vi "i2c_controller.vi"(5 "SDA in pin":refnum<k21>="SDA0", 6 "I2C clock divisor":u8=25, 7 "SCL out pin":refnum<k21>="SCL0", 8 "Read FIFO":refnum<k21>="I2C read 0", 9 "Write FIFO":refnum<k21>="I2C write 0", 10 "SDA out pin":refnum<k21>="SDA0", 11 "SCL in pin":refnum<k21>="SCL0") -> ()   [LabVIEW 2011]
uses:
  i2c_controller_state.ctl
  Common/i2c_status.ctl
  <vilib>/Platform/TimedLoop/XDataNode/timing_clust.ctl
  <vilib>/Platform/TimedLoop/XDataNode/nitl_modes.ctl
  <vilib>/Platform/TimedLoop/XDataNode/wakeup.ctl
  <vilib>/rvi/DataTransferAndStorage/Container/Common/niFpgaContainerExecOnDevCompGetState.vi
  <vilib>/rvi/FIFO/Fifo_Resource/nirvififoEmulationSetSize.vi
  <vilib>/rvi/DataTransferAndStorage/Container/Common/niFpgaContainerGetUniqueNameForEmu.vi
  <vilib>/rvi/interface/RandomDataEmulation/nirviRandomDataFPGAFIFO.vi
  <vilib>/rvi/interface/RandomDataEmulation/niFpgaRandomDataHandleErrors.vi
  <vilib>/rvi/eio/common/nirviEmuReportErrorAndStop.vi
  fpga_globals.vi
  <vilib>/Platform/TimedLoop/XDataNode/XDataNode.xnode
  <vilib>/rvi/DataTransferAndStorage/Container/XNode/niFpgaContainer.xnode
  <vilib>/rvi/FIFO/Fifo_Resource/niFpgaFifoEmulationRefIn.vi
  <vilib>/Platform/TimedLoop/XDataNode/XDNodeRunTimeDep.lvlib
panel:
  # "Clock"
  # "I2C bus I/O pins.  The input and output directions  may in general be distinct when an external buffer is used.  See output_buffer.vi"
  # "Data"
  # "Commands and data out to I2C"
  # "Status and data back from I2C"
  # "1/4 of the I2C bit time, in clock ticks"
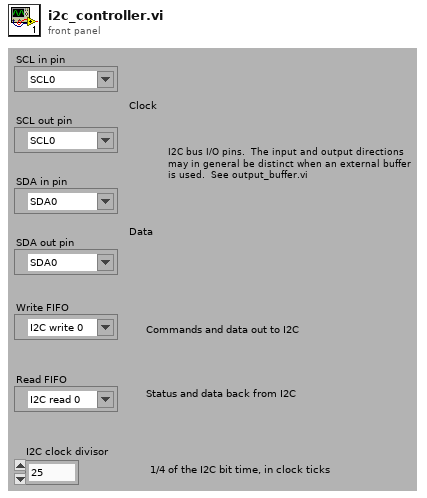
[diagram p1: front panel]
types:
  T1 = typedef "i2c_status.ctl" = enum8{"Invalid", "Command", "I2C start", "Trigger wait", "TX data wait", "Sequence", "Receive data", "I2C error", "Address NACK", "Data NACK", "SDA stuck", "SCL stuck", "Bad command"}
  T2 = typedef "i2c_controller_state.ctl" = enum8{"CMD wait", "start", "load", "address", "address ACK", "wait", "TX data", "TX data ACK", "stop wait", "stop", "RX data", "RX data 1", "RX data ACK", "Sequence arg load", "Trigger delay 1", "Trigger delay 2", "Trigger delay 3"}
  T3 = typedef "XDNodeRunTimeDep.lvlib/timing_clust.ctl" = cluster{"Expected End [f-1]":u64, "Actual End [f-1]":u64, "Finished Late? [f-1]":bool, "Expected End [i-1]":u64, "Actual End [i-1]":u64, "Finished Late? [i-1]":bool, "Expected Start [i]":u64, "Actual Start [i]":u64, "Expected Start [f]":u64, "Actual Start [f]":u64, "Source Name":string, "Structure Name":string, "Period":i64, "Deadline":i64, "Offset":i64, "Start":i64, "Priority":i32, "Timeout":i32, "Mode":T4, "Wakeup Reason":T5, "Error":errorcluster, "Source Type":string, "Secondary Source Type":string, "Global End Time":u64, "Global Start Time":u64, "Frame Duration":u64, "Iteration Duration":u64, "Assigned CPU":i32, "I/O Scan Engine Mode":u32}
  T4 = typedef "XDNodeRunTimeDep.lvlib/nitl_modes.ctl" = enum32{"No Change", "Process missed periods, maintain original phase", "Discard missed periods, maintain original phase", "Process missed periods, ignore original phase", "Discard missed periods, ignore original phase"}
  T5 = typedef "XDNodeRunTimeDep.lvlib/wakeup.ctl" = enum32{"Normal", "Aborted", "Asynchronous wakeup", "Timing source error", "Timed loop error", "Timeout"}
  T6 = typedef "i2c_command.ctl" = enum8{"invalid", "start_write", "start_read", "stop", "sequence"}
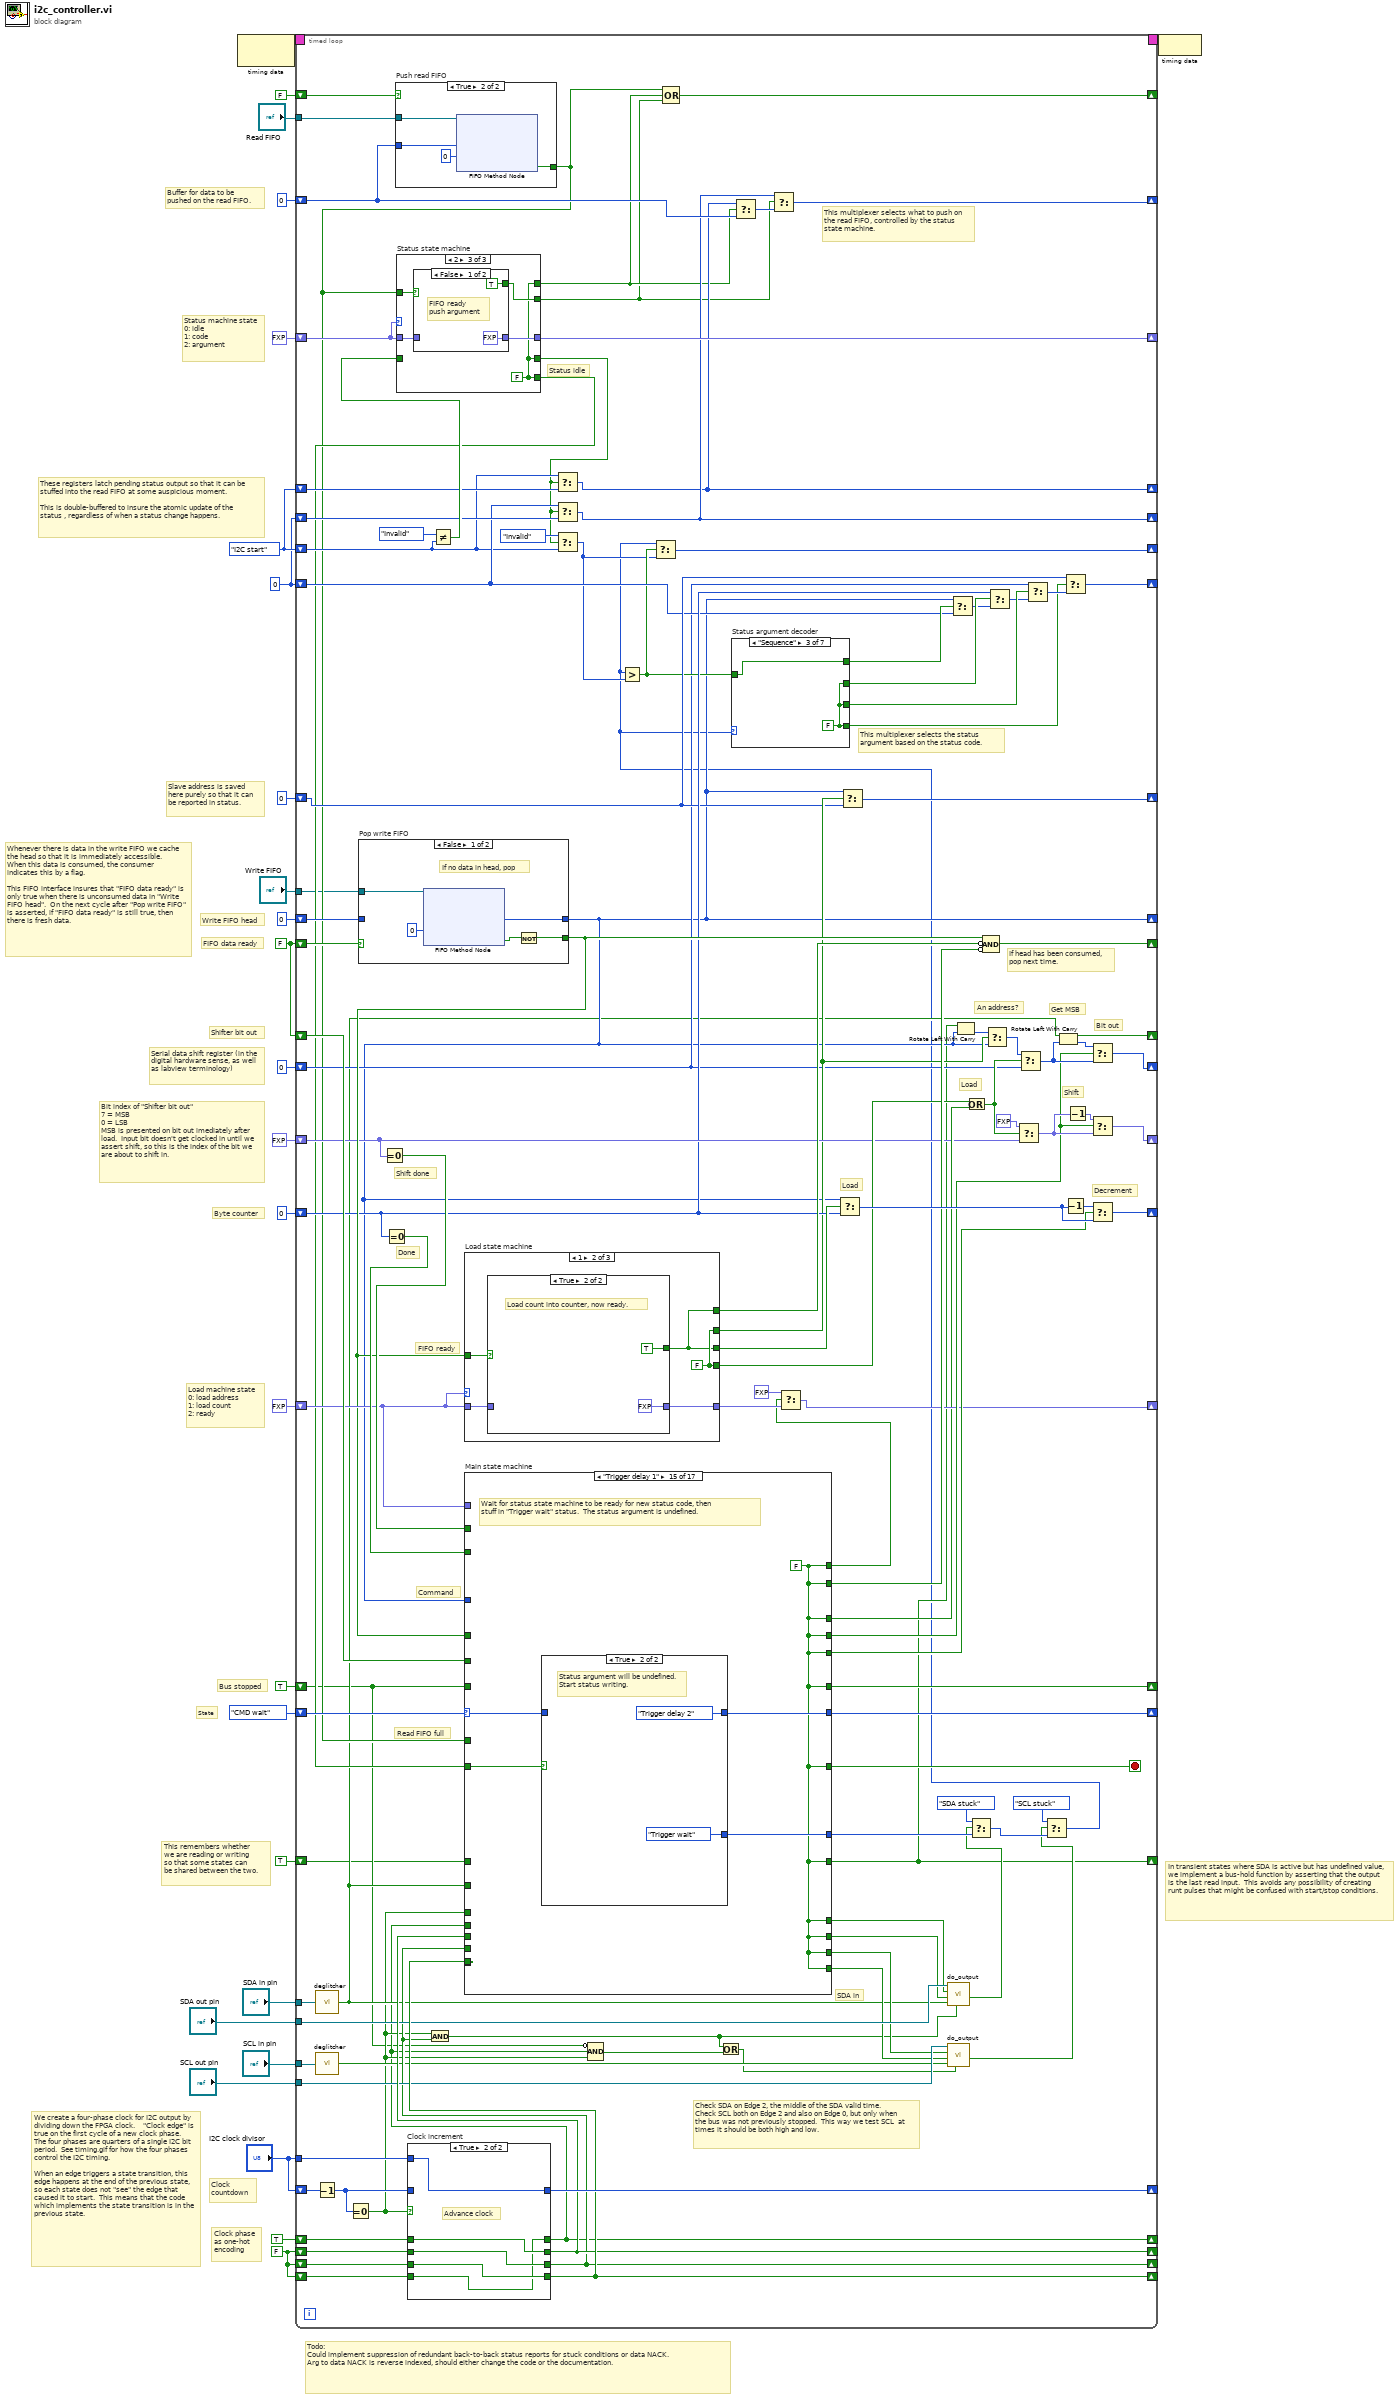
[diagram p0: block diagram]
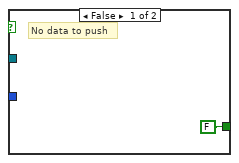
[diagram p2: hidden frame]
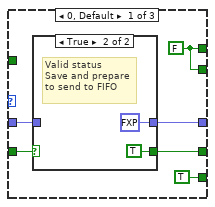
[diagram p3: hidden frame]
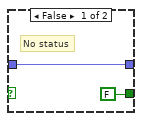
[diagram p4: hidden frame]
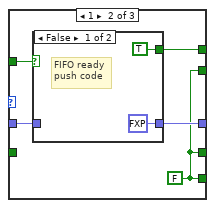
[diagram p5: hidden frame]
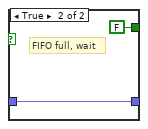
[diagram p6: hidden frame]
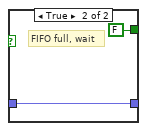
[diagram p7: hidden frame]
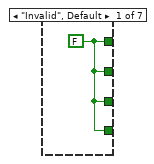
[diagram p8: hidden frame]
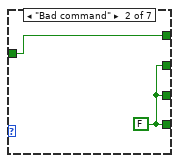
[diagram p9: hidden frame]
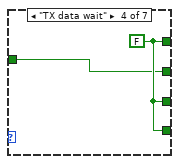
[diagram p10: hidden frame]
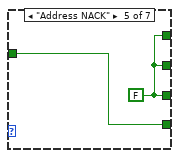
[diagram p11: hidden frame]
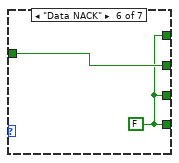
[diagram p12: hidden frame]
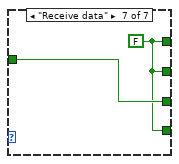
[diagram p13: hidden frame]
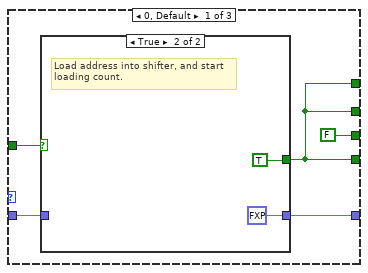
[diagram p14: hidden frame]
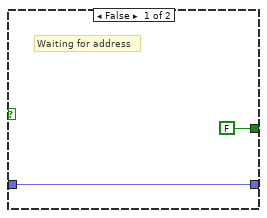
[diagram p15: hidden frame]
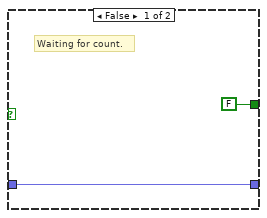
[diagram p16: hidden frame]
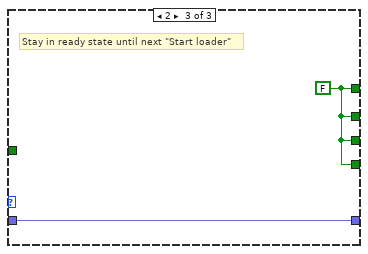
[diagram p17: hidden frame]
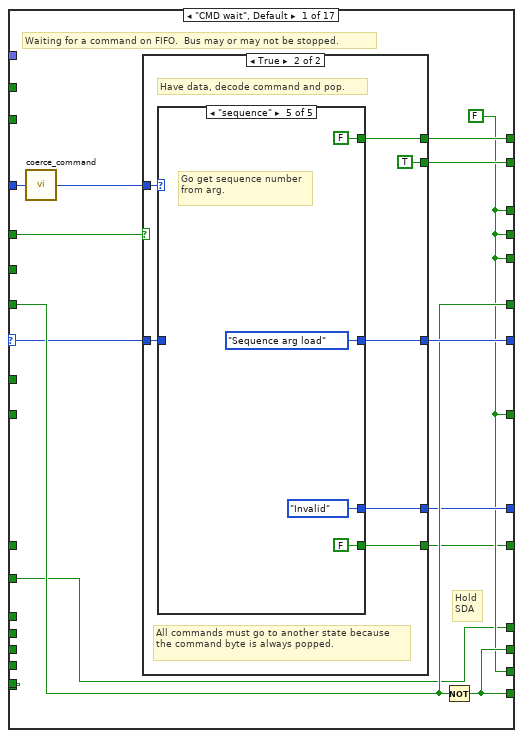
[diagram p18: hidden frame]
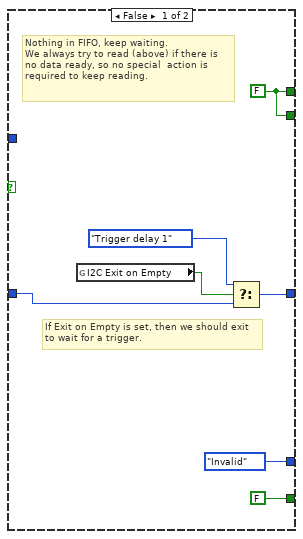
[diagram p19: hidden frame]
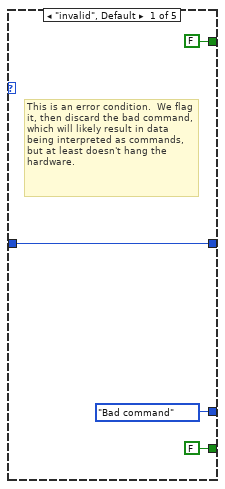
[diagram p20: hidden frame]
diagram:
  w10 = i2c_status."I2C start" ("Cluster")
  w9 = u8 0 ("Element")
  w15 = FALSE ("x = 0?")
  w19 = FALSE
  # "This remembers whether\nwe are reading or writing\nso that some states can\nbe shared between the two."
  # "In transient states where SDA is active but has undefined value, we implement a bus-hold function by asserting that the output is the last read input.  This avoids any possibility of creating runt pulses that might be confused with start/stop conditions."
  # "Buffer for data to be pushed on the read FIFO."
  # "Status machine state\n0: idle\n1: code\n2: argument"
  # "These registers latch pending status output so that it can be stuffed into the read FIFO at some auspicious moment.\n\nThis is double-buffered to insure the atomic update of the status , regardless of when a status change happens."
  # "Slave address is saved here purely so that it can be reported in status."
  # "Todo: \nCould implement suppression of redundant back-to-back status reports for stuck conditions or data NACK.\nArg to data NACK is reverse indexed, should either change the code or the documentation."
  # "Clock phase\nas one-hot\nencoding"
  # "Load machine state\n0: load address\n1: load count\n2: ready"
  # "Bus stopped"
  # "Shifter bit out"
  # "Byte counter"
  # "Serial data shift register (in the digital hardware sense, as well as labview terminology)"
  # "We create a four-phase clock for I2C output by dividing down the FPGA clock.    \"Clock edge\" is true on the first cycle of a new clock phase.  The four phases are quarters of a single I2C bit period.  See timing.gif for how the four phases control the I2C timing.\n\nWhen an edge triggers a state transition, this edge happens at the end of the previous state, so each state does not \"see\" the edge that caused it to start.  This means that the code which implements the state transition is in the previous state."
  # "Whenever there is data in the write FIFO we cache the head so that it is immediately accessible.  When this data is consumed, the consumer indicates this by a flag.\n\nThis FIFO interface insures that \"FIFO data ready\" is only true when there is unconsumed data in \"Write FIFO head\".  On the next cycle after \"Pop write FIFO\" is asserted, if \"FIFO data ready\" is still true, then there is fresh data."
  # "FIFO data ready"
  # "Clock countdown"
  # "Write FIFO head"
  # "State"
  # "Bit index of \"Shifter bit out\"\n7 = MSB\n0 = LSB\nMSB is presented on bit out imediately after load.  Input bit doesn't get clocked in until we assert shift, so this is the index of the bit we are about to shift in."
  n1 = node-c288() -> (w26:T3)  [unwired: 1 in]
  n2 = timed-loop {
    timing: w26 -> [_]
    timing-out: [_] -> w25
    shift-right: [w125] -> _
    shift-left: fxp<+,3,3> 0.0 -> [w94]
    shift-right: [w59] -> _
    shift-left: u8 0 ("Element") -> [w122]
    shift-right: [w139] -> _
    shift-left: "I2C clock divisor" -> [w140]
    tunnel: "I2C clock divisor" -> [w138]
    shift-right: [w56] -> _
    shift-left: i2c_controller_state."CMD wait" ("Enum") -> [w124]
    shift-right: [w113] -> _
    shift-left: w19 -> [w115]
    shift-right: [w129] -> _
    shift-left: u8 0 ("I2C clock divisor") -> [w67]
    shift-right: [w132] -> _
    shift-left: u8 0 ("I2C clock divisor") -> [w93]
    shift-right: [w121] -> _
    shift-left: w19 -> [w116]
    shift-right: [w54] -> _
    shift-left: TRUE ("x = 0?") -> [w35]
    shift-right: [w110] -> _
    shift-left: fxp<+,2,2> 2.0 -> [w112]
    shift-right: [w36] -> _
    shift-left: TRUE ("x = 0?") -> [w98]
    shift-right: [w96] -> _
    shift-left: w15 -> [w99]
    shift-right: [w43] -> _
    shift-left: w15 -> [w100]
    shift-right: [w97] -> _
    shift-left: w15 -> [w101]
    tunnel: "SDA out pin" -> [w55]
    tunnel: "SCL out pin" -> [w51]
    shift-right: [w95] -> _
    shift-left: w10 -> [w73]
    shift-right: [w83] -> _
    shift-left: w9 -> [w74]
    shift-right: [w86] -> _
    shift-left: u8 0 ("Element") -> [w84]
    shift-right: [w77] -> _
    shift-left: fxp<+,2,2> 0.0 -> [w79]
    shift-right: [w65] -> _
    shift-left: w10 -> [w76]
    shift-right: [w66] -> _
    shift-left: w9 -> [w75]
    shift-right: [w72] -> _
    shift-left: FALSE -> [w71]
    shift-right: [w27] -> _
    shift-left: u8 0 ("Element") -> [w69]
    tunnel: "Write FIFO" -> [w58]
    tunnel: "Read FIFO" -> [w57]
    tunnel: "SDA in pin" -> [w53]
    tunnel: "SCL in pin" -> [w52]
    shift-right: [w29] -> _
    shift-left: TRUE ("x = 0?") -> [w30]
    stop <- w123 stop-if-true
    # "Check SDA on Edge 2, the middle of the SDA valid time.\nCheck SCL both on Edge 2 and also on Edge 0, but only when the bus was not previously stopped.  This way we test SCL  at times it should be both high and low."
    # "SDA in"
    # "Status idle"
    # "Read FIFO full"
    # "This multiplexer selects what to push on the read FIFO, controlled by the status state machine."
    # "This multiplexer selects the status argument based on the status code."
    # "FIFO ready"
    # "Command"
    # "Bit out"
    # "Shift done"
    # "Done"
    # "Decrement"
    # "Load"
    # "Shift"
    # "Load"
    # "Get MSB"
    # "An address?"
    # "If head has been consumed, pop next time."
    n3 = call "deglitcher.vi"("Pin"=w53) -> ("Result"=w38:bool)
    n4 = call "deglitcher.vi"("Pin"=w52) -> ("Result"=w39:bool)
    n5 = Decrement(x=w140) -> (x-1=w137:u8)
    n6 = Equal To 0?(x=w137) -> (x = 0?=w37:bool)
    n7 = case "Pop write FIFO" shown="False" w115 {
      selector: w115 -> [_ w555]
      tunnel: w122 -> [_ w556]
      tunnel: [w553 w556] -> w59
      tunnel: [w551 w555] -> w106
      tunnel: w58 -> [w550 _]
      frame False {
        # "If no data in head, pop"
        n8 = xnode ("FIFO Method Node")("Timeout"=0, "FIFO In"=w550) -> ("Element"=w553:u8, "Timed Out?"=w552:bool)  [unwired: 1 out]
        n9 = Not(x=w552) -> (.not. x?=w551:bool)
      }
      frame True {
        # "Data in head, do nothing"
      }
    }
    n10 = Equal To 0?(x=w94) -> (x = 0?=w117:bool)
    n11 = Equal To 0?(x=w93) -> (x = 0?=w118:bool)
    n12 = case "Push read FIFO" shown="True" w71 {
      tunnel: [FALSE ("Timed Out?") w144] -> w60
      tunnel: w69 -> [_ w143]
      tunnel: w57 -> [_ w142]
      frame False {
        # "No data to push"
      }
      frame True {
        n13 = xnode ("FIFO Method Node")("Element"=w143, "Timeout"=0, "FIFO In"=w142) -> ("Timed Out?"=w144:bool)  [unwired: 1 out]
      }
    }
    n14 = case "Clock increment" shown="True" w37 {
      tunnel: [w561 w566] -> w139
      tunnel: w138 -> [_ w566]
      tunnel: w137 -> [w561 _]
      tunnel: w98 -> [w560 w565]
      tunnel: w99 -> [w559 w564]
      tunnel: w100 -> [w558 w563]
      tunnel: w101 -> [w557 w562]
      tunnel: [w560 w562] -> w36
      tunnel: [w559 w565] -> w96
      tunnel: [w558 w564] -> w43
      tunnel: [w557 w563] -> w97
      frame False {
      }
      frame True {
        # "Advance clock"
      }
    }
    n15 = And(x=w37, y=w43) -> (x .and. y?=w34:bool)
    n16 = Not Equal?(x=i2c_status."Invalid" ("y"), y=w73) -> (x != y?=w78:bool)
    n17 = case "Status state machine" shown="2" w79 {
      tunnel: w79 -> [w148 w159 w168]
      tunnel: w78 -> [w151 _ _]
      tunnel: [w149 w156 w165] -> w64
      tunnel: [w150 w160 w169] -> w77
      tunnel: w60 -> [_ w158 w167]
      tunnel: [w147 w157 w165] -> w63
      tunnel: [w147 w156 w166] -> w62
      tunnel: [TRUE w156 w165] -> w61
      frame 0, Default {
        w147 = FALSE
        n18 = case shown="True" w151 {
          tunnel: [w153 fxp<+,2,2> 1.0] -> w150
          tunnel: [FALSE TRUE] -> w149
          tunnel: w148 -> [w153 _]
          frame False {
            # "No status"
          }
          frame True {
            # "Valid status\nSave and prepare\nto send to FIFO"
          }
        }
      }
      frame 1 {
        w156 = FALSE
        n19 = case shown="False" w158 {
          tunnel: [fxp<+,2,2> 2.0 w164] -> w160
          tunnel: w159 -> [_ w164]
          tunnel: [TRUE FALSE] -> w157
          frame False {
            # "FIFO ready\npush code"
          }
          frame True {
            # "FIFO full, wait"
          }
        }
      }
      frame 2 {
        w165 = FALSE
        n20 = case shown="False" w167 {
          tunnel: [fxp<+,2,2> 0.0 w173] -> w169
          tunnel: w168 -> [_ w173]
          tunnel: [TRUE FALSE] -> w166
          frame False {
            # "FIFO ready\npush argument"
          }
          frame True {
            # "FIFO full, wait"
          }
        }
      }
    }
    n21 = case "Load state machine" shown="1" w112 {
      tunnel: [w189 w199 w205] -> w111
      tunnel: w112 -> [w188 w198 w205]
      tunnel: [w187 w197 w206] -> w87
      tunnel: [FALSE ("x = 0?") w196 w206] -> w107
      tunnel: w106 -> [w190 w200 _]
      tunnel: [w187 w197 w206] -> w103
      tunnel: [w187 w196 w206] -> w102
      frame 0, Default {
        n22 = case shown="True" w190 {
          tunnel: [w193 fxp<+,2,2> 1.0] -> w189
          tunnel: [FALSE ("x = 0?") TRUE ("x = 0?")] -> w187
          tunnel: w188 -> [w193 _]
          frame False {
            # "Waiting for address"
          }
          frame True {
            # "Load address into shifter, and start\nloading count."
          }
        }
      }
      frame 1 {
        w197 = FALSE ("x = 0?")
        n23 = case shown="True" w200 {
          tunnel: [w202 fxp<+,2,2> 2.0] -> w199
          tunnel: [FALSE ("x = 0?") TRUE ("x = 0?")] -> w196
          tunnel: w198 -> [w202 _]
          frame False {
            # "Waiting for count."
          }
          frame True {
            # "Load count into counter, now ready."
          }
        }
      }
      frame 2 {
        w206 = FALSE ("x = 0?")
        # "Stay in ready state until next \"Start loader\""
      }
    }
    n24 = case "Main state machine" shown="\"Trigger delay 1\"" w124 {
      selector: w124 -> [w215 w263 w279 w307 w335 w355 w397 w419 w440 w460 w468 w487 w498 w521 w533 _ w547]
      tunnel: [w220 w266 w286 w311 w337 w357 w401 w418 w441 w462 w470 w489 w503 w523 w535 i2c_controller_state."Trigger delay 3" ("Enum") w547] -> w56
      tunnel: w106 -> [w218 _ _ _ _ w344 _ _ _ _ _ _ _ w519 _ _ _]
      tunnel: w59 -> [w211 _ _ _ _ _ _ _ _ _ _ _ _ _ _ _ _]
      tunnel: [w209 w257 w278 w306 w325 w341 w386 w416 w431 w448 w473 w480 w492 w515 w531 w541 w546] -> w123
      tunnel: [w219 w265 w275 w297 w325 w347 w387 w415 w431 w448 w466 w488 w493 w516 w531 w541 w545] -> w49
      tunnel: [w219 w265 w275 w297 TRUE ("x = 0?") w347 w387 TRUE ("x = 0?") TRUE ("x = 0?") TRUE ("x = 0?") w466 w488 w493 w516 w531 w541 w545] -> w40
      tunnel: [w209 w257 w278 w306 w325 w354 w386 w416 w431 w448 w473 w480 w492 w515 w531 w541 w545] -> w104
      tunnel: [w209 w257 w278 w303 w325 w341 w394 w417 w431 w448 w473 w480 w492 w515 w531 w541 w545] -> w120
      tunnel: [w209 w257 w278 w306 w325 w341 w390 w416 w439 w448 w473 w480 w492 w515 w531 w541 w545] -> w119
      tunnel: [w213 w257 w278 w306 w325 w346 w386 w416 w431 w448 w473 w480 w492 w514 w531 w541 w545] -> w114
      tunnel: w118 -> [_ _ _ _ _ w348 _ _ _ _ w465 _ _ _ _ _ _]
      tunnel: w117 -> [_ _ _ w301 _ _ w392 w424 _ _ _ _ _ _ _ _ _]
      tunnel: w116 -> [_ _ _ w299 _ _ w389 _ _ _ _ _ _ _ _ _ _]
      tunnel: w37 -> [_ w261 w287 w305 w332 w353 w396 w425 w436 w457 w477 w485 w504 _ _ _ _]
      tunnel: w35 -> [w217 w264 w280 _ _ _ _ _ _ _ _ w481 w497 w517 _ _ _]
      tunnel: [w217 w264 w285 w306 w325 w341 w386 w416 w431 w448 w473 w481 w502 w517 w531 w541 w545] -> w54
      tunnel: w112 -> [_ w259 _ _ _ _ _ _ _ _ _ _ _ _ _ _ _]
      tunnel: [w216 w257 w278 w306 w325 w341 w386 w416 w431 w448 w473 w480 w492 w515 w531 w541 w545] -> w108
      tunnel: [w214 w262 w282 w310 w331 w356 w400 w426 w435 w456 w476 w486 w500 w524 w536 w544 w549] -> _
      tunnel: w97 -> [w214 w262 w282 w310 w331 w356 w400 w426 w435 w456 w476 w486 w500 w524 w536 w544 w549]
      tunnel: w43 -> [_ _ _ w308 w330 _ w398 w423 w433 w455 w475 _ _ _ _ _ _]
      tunnel: w96 -> [_ _ _ w309 w336 _ w399 w430 _ w461 w478 _ _ _ _ _ _]
      tunnel: w36 -> [_ w260 w283 w304 _ w352 w395 _ _ _ _ w484 w499 _ _ _ _]
      tunnel: w38 -> [w207 w255 _ _ w333 w340 _ _ _ w458 _ w479 _ w513 _ _ _]
      tunnel: [w212 i2c_status."Invalid" ("Cluster") i2c_status."Invalid" ("Cluster") i2c_status."Invalid" ("Cluster") w326 w350 i2c_status."Invalid" ("Cluster") i2c_status."Invalid" ("Cluster") w437 w451 i2c_status."Invalid" ("Cluster") i2c_status."Invalid" ("Cluster") i2c_status."Invalid" ("Cluster") w522 w534 i2c_status."Invalid" ("Cluster") i2c_status."Invalid" ("Cluster")] -> w48
      tunnel: w61 -> [_ _ _ _ _ w343 _ _ _ _ _ _ _ w518 w532 _ w546]
      tunnel: w60 -> [_ _ _ _ _ _ _ _ _ _ _ _ _ _ _ _ _]
      tunnel: [w207 w255 w277 w299 w325 w340 w389 w415 w431 w448 w465 w479 w495 w513 w531 w541 w545] -> w50
      tunnel: [w209 w257 w276 w298 w324 w341 w388 w429 w433 w450 w474 w480 w494 w515 w531 w541 w545] -> w41
      tunnel: w30 -> [_ w256 w274 w296 w322 w345 _ w427 w438 _ w471 _ _ _ _ _ _]
      tunnel: [w208 w256 w274 w296 w322 w345 w386 w427 w438 w448 w471 w480 w492 w515 w531 w541 w545] -> w29
      frame "CMD wait", Default {
        w209 = FALSE ("x = 0?")
        # "Hold\nSDA"
        # "Waiting for a command on FIFO.  Bus may or may not be stopped."
        n25 = call "coerce_command.vi"("U8 code"=w211) -> ("Command"=w210:T6)
        n26 = case shown="True" w218 {
          tunnel: [w223 w234] -> w220
          tunnel: w210 -> [_ w233]
          tunnel: [w227 w232] -> w216
          tunnel: w215 -> [w224 w231]
          tunnel: [w227 TRUE ("x = 0?")] -> w213
          tunnel: [i2c_status."Invalid" ("Cluster") w230] -> w212
          tunnel: [FALSE ("x = 0?") w228] -> w208
          frame False {
            w227 = FALSE ("x = 0?")
            # "If Exit on Empty is set, then we should exit to wait for a trigger."
            # "Nothing in FIFO, keep waiting.\nWe always try to read (above) if there is no data ready, so no special  action is required to keep reading."
            n27 = global read "fpga_globals.vi" "I2C Exit on Empty"() -> (w225:bool)
            n28 = Select(t=i2c_controller_state."Trigger delay 1" ("Enum"), s=w225, f=w224) -> (s? t:f=w223:T2)
          }
          frame True {
            # "All commands must go to another state because the command byte is always popped."
            # "Have data, decode command and pop."
            n29 = case shown="\"sequence\"" w233 {
              tunnel: [w238 i2c_controller_state."load" ("Enum") i2c_controller_state."load" ("Enum") i2c_controller_state."stop wait" ("Enum") i2c_controller_state."Sequence arg load" ("Enum")] -> w234
              tunnel: [FALSE ("x = 0?") TRUE ("x = 0?") TRUE ("x = 0?") FALSE ("x = 0?") FALSE ("x = 0?")] -> w232
              tunnel: w231 -> [w238 _ _ _ _]
              tunnel: [i2c_status."Bad command" ("Cluster") i2c_status."Invalid" ("Cluster") i2c_status."Invalid" ("Cluster") i2c_status."Invalid" ("Cluster") i2c_status."Invalid" ("Cluster")] -> w230
              tunnel: [FALSE ("x = 0?") FALSE ("x = 0?") TRUE ("x = 0?") FALSE ("x = 0?") FALSE ("x = 0?")] -> w228
              frame "invalid", Default {
                # "This is an error condition.  We flag it, then discard the bad command, which will likely result in data being interpreted as commands, but at least doesn't hang the hardware."
              }
              frame "start_write" {
                # "Start load state machine."
              }
              frame "start_read" {
                # "Start load state machine."
              }
              frame "stop" {
                # "Transition to \"stop wait\" state."
              }
              frame "sequence" {
                # "Go get sequence number from arg."
              }
            }
          }
        }
        n30 = Not(x=w217) -> (.not. x?=w219:bool)
      }
      frame "load" {
        w257 = FALSE ("x = 0?")
        # "Loading FIFO args for TX/RX, wait until complete."
        n31 = case shown="2" w259 {
          tunnel: [w267 w271] -> w266
          tunnel: w263 -> [w267 w268]
          tunnel: w261 -> [_ w270]
          tunnel: w260 -> [_ w269]
          frame 0, Default {
            # "Waiting for load to finish."
          }
          frame 2 {
            # "Args loaded, go to start state on phase 0."
            n32 = And(x=w270, y=w269) -> (x .and. y?=w272:bool)
            n33 = Select(t=i2c_controller_state."start" ("Enum"), s=w272, f=w268) -> (s? t:f=w271:T2)
          }
        }
        n34 = Not(x=w264) -> (.not. x?=w265:bool)
      }
      frame "start" {
        w275 = TRUE ("x = 0?")
        w278 = FALSE ("x = 0?")
        # "Sending start bit for TX/RX"
        n35 = And(x=w287, y=w283) -> (x .and. y?=w284:bool)
        n36 = case shown="True" w284 {
          tunnel: [w291 i2c_controller_state."address" ("Enum")] -> w286
          tunnel: [w292 FALSE ("x = 0?")] -> w285
          tunnel: w283 -> [w289 _]
          tunnel: w282 -> [w290 _]
          tunnel: [w289 w293] -> w277
          tunnel: [w288 w293] -> w276
          tunnel: w280 -> [w292 _]
          tunnel: w279 -> [w291 _]
          frame False {
            # "Still sending"
            # "SDA high only in phase 0\nSCL low only in phase 3"
            n37 = Not(x=w290) -> (.not. x?=w288:bool)
          }
          frame True {
            w293 = FALSE
            # "Phase 0 edge"
            # "Now not stoppped."
            # "Next state  address"
          }
        }
      }
      frame "address" {
        w297 = TRUE ("x = 0?")
        w306 = FALSE ("x = 0?")
        # "SCL high in phase 1,2"
        # "SDA is shifter out"
        # "Sending I2C address"
        n38 = And(x=w305, y=w304) -> (x .and. y?=w302:bool)
        n39 = Or(x=w309, y=w308) -> (x .or. y?=w298:bool)
        n40 = case shown="True" w302 {
          tunnel: [w313 w317] -> w311
          tunnel: w307 -> [w313 w314]
          tunnel: [FALSE w315] -> w303
          tunnel: w301 -> [_ w316]
          frame False {
            # "Not phase 0 edge, do nothing"
          }
          frame True {
            # "Phase 0 edge"
            n41 = case shown="True" w316 {
              tunnel: [w319 i2c_controller_state."address ACK" ("Enum")] -> w317
              tunnel: [TRUE ("x = 0?") FALSE ("x = 0?")] -> w315
              tunnel: w314 -> [w319 _]
              frame False {
                # "Waiting for shift to finish.\nShift next bit."
              }
              frame True {
                # "Shift done"
                # "Next state check ACK"
              }
            }
          }
        }
      }
      frame "address ACK" {
        w325 = FALSE ("x = 0?")
        # "Test SDA on edge 2 (middle of SCL pulse)"
        # "SCL high in phase 1,2"
        # "Checking ACK for address\n\nIdentical to the TX data case, except that we assert a different status on NACK"
        n42 = And(x=w332, y=w331) -> (x .and. y?=w334:bool)
        n43 = Or(x=w336, y=w330) -> (x .or. y?=w324:bool)
        n44 = Compound Arithmetic op=AND(w333, w332, w330) -> (w327:bool)
        n45 = case shown="True" w334 {
          tunnel: [w338 i2c_controller_state."wait" ("Enum")] -> w337
          tunnel: w335 -> [w338 _]
          frame False {
            # "Not phase 3 edge, do nothing"
          }
          frame True {
            # "Phase 3 edge (end of SCL pulse)\n\nContinue to wait state in this bit period to get data ready before phase 0 edge."
          }
        }
        n46 = Select(t=i2c_status."Address NACK" ("Cluster"), s=w327, f=i2c_status."Invalid" ("Cluster")) -> (s? t:f=w326:T1)
      }
      frame "wait" {
        w347 = TRUE ("x = 0?")
        w341 = FALSE ("x = 0?")
        # "Hold SDA"
        # "We normally enter this state on phase 3 of the previous bit period, after the clock for the ACK ends.  If the next byte is ready, then it will transmit on the immediately following clock 0 edge.  If the data is not ready, then we wait for whole bit periods (holding SCL low)  to keep the phase correct.  Similarly, on read, we wait for the status machine to finish\nwriting."
        # "Waiting to be ready for next data read/write.  This is where we check whether all data as been written/read."
        n47 = And(x=w353, y=w352) -> (x .and. y?=w349:bool)
        n48 = Select(t=w343, s=w345, f=w344) -> (s? t:f=w342:bool)
        n49 = And(x=w342, y=w349) -> (x .and. y?=w351:bool)
        n50 = case shown="True" w348 {
          tunnel: [w365 w383] -> w357
          tunnel: w355 -> [w364 w380]
          tunnel: [w363 w379] -> w354
          tunnel: w351 -> [w362 _]
          tunnel: [w361 i2c_status."Invalid" ("Cluster")] -> w350
          tunnel: w349 -> [w360 w381]
          tunnel: w345 -> [w359 _]
          tunnel: [w358 w379] -> w346
          frame False {
            # "Not done with read/write op"
            n51 = case shown="True" w362 {
              tunnel: [w371 w374] -> w365
              tunnel: [w366 TRUE ("x = 0?")] -> w363
              tunnel: w364 -> [w371 _]
              tunnel: [w368 i2c_status."Invalid" ("Cluster")] -> w361
              tunnel: w360 -> [w367 _]
              tunnel: w359 -> [_ w372]
              tunnel: [w366 w373] -> w358
              frame False {
                w366 = FALSE ("x = 0?")
                # "Only report wait state if edge 0\npasses."
                # "Still waiting"
                n52 = Select(t=i2c_status."TX data wait" ("Cluster"), s=w367, f=i2c_status."Invalid" ("Cluster")) -> (s? t:f=w368:T1)
              }
              frame True {
                # "Phase 0 edge and data is ready.  Load shift register and pop FIFO, go to transmit.  If reading, we just load the FIFO (to reset the bit counter) and don't pop."
                n53 = Select(t=i2c_controller_state."RX data" ("Enum"), s=w372, f=i2c_controller_state."TX data" ("Enum")) -> (s? t:f=w374:T2)
                n54 = Not(x=w372) -> (.not. x?=w373:bool)
              }
            }
          }
          frame True {
            w379 = FALSE ("x = 0?")
            # "If done with read/write, go to \"CMD wait\"  on edge 0."
            n55 = case shown="True" w381 {
              tunnel: [w384 i2c_controller_state."CMD wait" ("Enum")] -> w383
              tunnel: w380 -> [w384 _]
              frame False {
              }
              frame True {
              }
            }
          }
        }
      }
      frame "TX data" {
        w387 = TRUE ("x = 0?")
        w386 = FALSE ("x = 0?")
        # "SCL high in phase 1,2"
        # "SDA is shifter out"
        # "Sending I2C data"
        n56 = And(x=w396, y=w395) -> (x .and. y?=w393:bool)
        n57 = Or(x=w399, y=w398) -> (x .or. y?=w388:bool)
        n58 = case shown="True" w393 {
          tunnel: [w403 w408] -> w401
          tunnel: w397 -> [w403 w406]
          tunnel: [w402 w404] -> w394
          tunnel: w392 -> [_ w407]
          tunnel: [w402 w405] -> w390
          frame False {
            w402 = FALSE
            # "Not phase 0 edge, do nothing"
          }
          frame True {
            # "Phase 0 edge"
            n59 = case shown="True" w407 {
              tunnel: [w410 i2c_controller_state."TX data ACK" ("Enum")] -> w408
              tunnel: [TRUE ("x = 0?") FALSE ("x = 0?")] -> w404
              tunnel: w406 -> [w410 _]
              tunnel: [FALSE ("x = 0?") TRUE ("x = 0?")] -> w405
              frame False {
                # "Waiting for shift to finish.\nShift next bit."
              }
              frame True {
                # "Shift done, decrement count and check ACK."
              }
            }
          }
        }
      }
      frame "RX data" {
        w415 = FALSE ("x = 0?")
        w416 = FALSE ("x = 0?")
        # "Edge 2 &  shift done: Shift in last bit and go to \"RX data 1\" state to save the byte we just read."
        # "SCL high in phase 1,2"
        # "SDA is not driven\n(inactive)"
        # "Receiving I2C data\nSDA input data is always shifted into shifter, no matter whether we are reading or writing.  On read, we clock at edge 2, the middle of the SCL clock period."
        n60 = And(x=w425, y=w423) -> (x .and. y?=w417:bool)
        n61 = Or(x=w430, y=w423) -> (x .or. y?=w429:bool)
        n62 = And(x=w424, y=w417) -> (x .and. y?=w420:bool)
        n63 = Select(t=i2c_controller_state."RX data 1" ("Enum"), s=w420, f=w419) -> (s? t:f=w418:T2)
      }
      frame "RX data 1" {
        w431 = FALSE ("x = 0?")
        # "SCL high in phase 2"
        # "SDA is not driven\n(inactive)"
        # "Phase 2 of the last bit period in a received byte.\nThis finishes out receiving the byte and also delays us past edge 3 of the last bit so that \"RX data ACK\" doesn't clock off of the wrong edge 3."
        n64 = And(x=w436, y=w435) -> (x .and. y?=w432:bool)
        n65 = case shown="False" w432 {
          tunnel: [w444 i2c_controller_state."RX data ACK" ("Enum")] -> w441
          tunnel: w440 -> [w444 _]
          tunnel: [FALSE TRUE ("x = 0?")] -> w439
          tunnel: [i2c_status."Invalid" ("Cluster") i2c_status."Receive data" ("Cluster")] -> w437
          frame False {
            # "Not phase 3 edge, keep going."
          }
          frame True {
            # "Edge 3 : decrement count, put data into status and go generate ACK."
          }
        }
      }
      frame "TX data ACK" {
        w448 = FALSE ("x = 0?")
        # "Test SDA on edge 2 (middle of SCL pulse)"
        # "SCL high in phase 1,2"
        # "Checking ACK for data\n\nIdentical to the address case, except that we assert a different status on NACK."
        n66 = And(x=w457, y=w456) -> (x .and. y?=w459:bool)
        n67 = Or(x=w461, y=w455) -> (x .or. y?=w450:bool)
        n68 = case shown="True" w459 {
          tunnel: [w463 i2c_controller_state."wait" ("Enum")] -> w462
          tunnel: w460 -> [w463 _]
          frame False {
            # "Not phase 3 edge, do nothing"
          }
          frame True {
            # "Phase 3 edge (end of SCL pulse)\n\nContinue to TX wait state in this bit period to allow shift register to load before phase 0 edge."
          }
        }
        n69 = Compound Arithmetic op=AND(w458, w457, w455) -> (w452:bool)
        n70 = Select(t=i2c_status."Data NACK" ("Cluster"), s=w452, f=i2c_status."Invalid" ("Cluster")) -> (s? t:f=w451:T1)
      }
      frame "RX data ACK" {
        w466 = TRUE ("x = 0?")
        w473 = FALSE ("x = 0?")
        # "Phase 3 edge (end of SCL pulse)\n\nContinue on to wait state in this bit period to allow data setup before phase 0 edge."
        # "SCL high in phase 1,2"
        # "Generate ACK/NACK for receive data.  This state runs from phase 3 of the last data bit period to phase 3 of the ACK.  We figure we regain control of the bus at the start of this state, so we assert the ACK/NACK for the duration of the state.  We leave this state on edge 3, so the hold timing is the responsibility of the wait state. \n\nThe read ACK is only quasi-symmetric with write ACK, since the convention is that it is used to terminate a transfer, rather than to indicate a failure condition.   We  ACK every byte but the last.   If we can't complete the read because the host read FIFO is full, then we block in the \"wait\" state."
        n71 = And(x=w477, y=w476) -> (x .and. y?=w467:bool)
        n72 = Or(x=w478, y=w475) -> (x .or. y?=w474:bool)
        n73 = Select(t=i2c_controller_state."wait" ("Enum"), s=w467, f=w468) -> (s? t:f=w470:T2)
      }
      frame "stop wait" {
        w480 = FALSE ("x = 0?")
        # "Wait for edge 0 before starting stop bit."
        n74 = And(x=w485, y=w484) -> (x .and. y?=w483:bool)
        n75 = case shown="True" w483 {
          tunnel: [w490 i2c_controller_state."stop" ("Enum")] -> w489
          tunnel: w487 -> [w490 _]
          frame False {
            # "Wait for edge 0"
          }
          frame True {
            # "Start stopping on edge 0"
          }
        }
        n76 = Not(x=w481) -> (.not. x?=w488:bool)
      }
      frame "stop" {
        w493 = TRUE ("x = 0?")
        w492 = FALSE ("x = 0?")
        # "Sending stop bit"
        n77 = And(x=w504, y=w499) -> (x .and. y?=w501:bool)
        n78 = case shown="False" w501 {
          tunnel: [w509 i2c_controller_state."CMD wait" ("Enum")] -> w503
          tunnel: [w508 TRUE ("x = 0?")] -> w502
          tunnel: w500 -> [w507 _]
          tunnel: [w505 w510] -> w494
          tunnel: [w507 w510] -> w495
          tunnel: w499 -> [w506 _]
          tunnel: w498 -> [w509 _]
          tunnel: w497 -> [w508 _]
          frame False {
            # "Still sending"
            # "SDA high only in phase 3\nSCL low only in phase 0"
            n79 = Not(x=w506) -> (.not. x?=w505:bool)
          }
          frame True {
            w510 = TRUE ("x = 0?")
            # "Phase 0 edge"
            # "Now  stopped."
          }
        }
      }
      frame "Sequence arg load" {
        w515 = FALSE ("x = 0?")
        # "Wait for argument byte (sequence number) to load and for status state machine to be ready for new status code.   All this command does is generate a status return."
        n80 = And(x=w519, y=w518) -> (x .and. y?=w520:bool)
        n81 = case shown="True" w520 {
          tunnel: [w526 i2c_controller_state."CMD wait" ("Enum")] -> w523
          tunnel: [i2c_status."Invalid" ("Cluster") i2c_status."Sequence" ("Cluster")] -> w522
          tunnel: w521 -> [w526 _]
          tunnel: [FALSE ("x = 0?") TRUE ("x = 0?")] -> w514
          frame False {
            # "Not loaded yet."
          }
          frame True {
            # "Load argument into status and start status writing."
          }
        }
        n82 = Not(x=w517) -> (.not. x?=w516:bool)
      }
      frame "Trigger delay 1" {
        w531 = FALSE ("x = 0?")
        # "Wait for status state machine to be ready for new status code, then\nstuff in \"Trigger wait\" status.  The status argument is undefined."
        n83 = case shown="True" w532 {
          tunnel: [w537 i2c_controller_state."Trigger delay 2" ("Enum")] -> w535
          tunnel: [i2c_status."Invalid" ("Cluster") i2c_status."Trigger wait" ("Cluster")] -> w534
          tunnel: w533 -> [w537 _]
          frame False {
            # "Not ready  yet."
          }
          frame True {
            # "Status argument will be undefined.  Start status writing."
          }
        }
      }
      frame "Trigger delay 2" {
        w541 = FALSE ("x = 0?")
        # "Give status state machine a chance to start before we test whether it is done."
      }
      frame "Trigger delay 3" {
        w545 = FALSE ("x = 0?")
        # "Wait for status to finish writing"
      }
    }
    n84 = Select(t=w73, s=w64, f=w76) -> (s? t:f=w65:T1)
    n85 = Select(t=w74, s=w64, f=w75) -> (s? t:f=w66:u8)
    n86 = Select(t=i2c_status."Invalid", s=w64, f=w73) -> (s? t:f=w31:T1)
    n87 = Compound Arithmetic op=AND(invert w35, w36, w37) -> (w33:bool)
    n88 = Compound Arithmetic op=OR(w60, w63, w62) -> (w72:bool)
    n89 = Or(x=w34, y=w33) -> (x .or. y?=w32:bool)
    n90 = Select(t=w65, s=w63, f=w69) -> (s? t:f=w70:u8)
    n91 = Select(t=w66, s=w62, f=w70) -> (s? t:f=w27:u8)
    n92 = Select(t=fxp<+,2,2> 0.0, s=w108, f=w111) -> (s? t:f=w110:fxp<+,2,2>)
    n93 = Select(t=w59, s=w107, f=w93) -> (s? t:f=w133:u8)
    n94 = Select(t=w59, s=w87, f=w84) -> (s? t:f=w86:u8)
    n95 = call "do_output.vi"("In clock"=w34, "In value"=w38, "Out active"=w49, "Out value"=w50, "Out pin"=w55) -> ("Stuck"=w46:bool)  [unwired: 6 in]
    n96 = call "do_output.vi"("In clock"=w32, "In value"=w39, "Out active"=w40, "Out value"=w41, "Out pin"=w51) -> ("Stuck"=w42:bool)  [unwired: 6 in]
    n97 = Rotate Left With Carry(2:w59, 3:w29) -> (0:w135:u8)  [unwired: 1 out]
    n98 = Or(x=w103, y=w104) -> (x .or. y?=w105:bool)
    n99 = Select(t=i2c_status."SDA stuck", s=w46, f=w48) -> (s? t:f=w44:T1)
    n100 = Compound Arithmetic op=AND(w106, invert w102, invert w114) -> (w113:bool)
    n101 = Select(t=w135, s=w87, f=w59) -> (s? t:f=w136:u8)
    n102 = Select(t=fxp<+,3,3> 7.0, s=w105, f=w94) -> (s? t:f=w126:fxp<+,3,3>)
    n103 = Select(t=w136, s=w105, f=w67) -> (s? t:f=w130:u8)
    n104 = Select(t=i2c_status."SCL stuck", s=w42, f=w44) -> (s? t:f=w28:T1)
    n105 = Greater?(x=w28, y=w31) -> (0:w68:bool)
    n106 = Select(t=w28, s=w68, f=w31) -> (s? t:f=w95:T1)
    n107 = case "Status argument decoder" shown="\"Sequence\"" w28 {
      tunnel: [w174 w176 w178 w179 w182 w184 w185] -> w92
      tunnel: [w174 w176 w178 w180 w182 w183 w186] -> w91
      tunnel: [w174 w175 w177 w180 w182 w183 w185] -> w88
      tunnel: [w174 w176 w178 w180 w181 w183 w185] -> w82
      tunnel: w68 -> [_ w175 w177 w179 w181 w184 w186]
      frame "Invalid", Default {
        w174 = FALSE
      }
      frame "Bad command" {
        w176 = FALSE
      }
      frame "Sequence" {
        w178 = FALSE
      }
      frame "TX data wait" {
        w180 = FALSE
      }
      frame "Address NACK" {
        w182 = FALSE
      }
      frame "Data NACK" {
        w183 = FALSE
      }
      frame "Receive data" {
        w185 = FALSE
      }
    }
    n108 = Select(t=w59, s=w88, f=w74) -> (s? t:f=w89:u8)
    n109 = Select(t=w93, s=w92, f=w89) -> (s? t:f=w90:u8)
    n110 = Select(t=w67, s=w91, f=w90) -> (s? t:f=w85:u8)
    n111 = Rotate Left With Carry(2:w130, 3:w38) -> (0:w131:u8, 1:w121:bool)
    n112 = Select(t=w84, s=w82, f=w85) -> (s? t:f=w83:u8)
    n113 = Decrement(x=w133) -> (x-1=w134:u8)
    n114 = Decrement(x=w126) -> (x-1=w127:fxp<+,3,3>)
    n115 = Select(t=w131, s=w120, f=w130) -> (s? t:f=w129:u8)
    n116 = Select(t=w127, s=w120, f=w126) -> (s? t:f=w125:fxp<+,3,3>)
    n117 = Select(t=w134, s=w119, f=w133) -> (s? t:f=w132:u8)
  }
  n118 = node-c288(w25) -> ()
